vi "Label_Ranking_Average_PS.vi"(7 "Type y_true":T1(ring), 8 "error in (no error)":errorcluster caption="entrée d'erreur (pas d'erreur)", 9 "y_score":string[][](array[string]), 10 "y_true":string[][](array[string]), 11 "label_ranking_average_precision_score":cluster{"sample_weight":dbl[]}) -> (0 "error out":errorcluster caption="sortie d'erreur", 3 "Score":string)   [LabVIEW 2020]
doc: "Compute ranking-based average precision\n\nLabel ranking average precision (LRAP) is the average over each ground truth label assigned to each sample, of the ratio of true vs. total labels with lower score.\n\nThis metric is used in multilabel ranking problem, where the goal is to give better rank to the labels associated to each sample.\n\nThe obtained score is always strictly greater than 0 and the best value is 1.\n\n\n\nParameters : \n\n- y_true : array or sparse matrix, shape = [n_samples, n_labels]\nTrue binary labels in binary indicator format.\n\n- y_score : array, shape = [n_samples, n_labels]\nTarget scores, can either be probability estimates of the positive class, confidence values, or non-thresholded measure of decisions (as returned by “decision_function” on some classifiers).\n\n- sample_weight : array-like of shape (n_samples,), default=None\nSample weights.\n\n\nReturns : \n\n- score : float"
uses:
  Label_Ranking_Average_PS.lvclass
panel:
  out "Label_Ranking_Average_PS en entrée":refnum<class "Label_Ranking_Average_PS.lvclass">
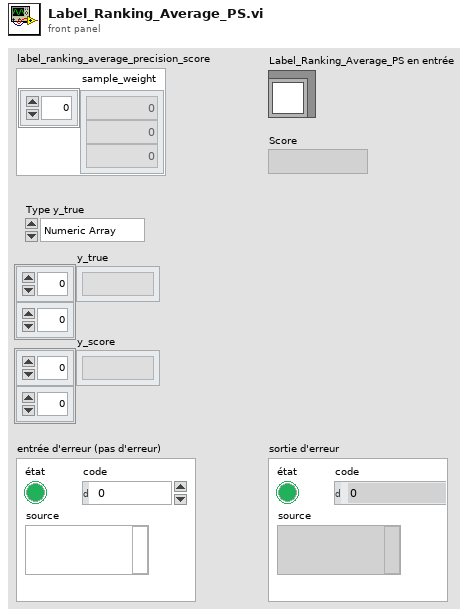
[diagram p1: front panel]
types:
  T1 = enum16{"Numeric Array", "String Array", "Sparse"}
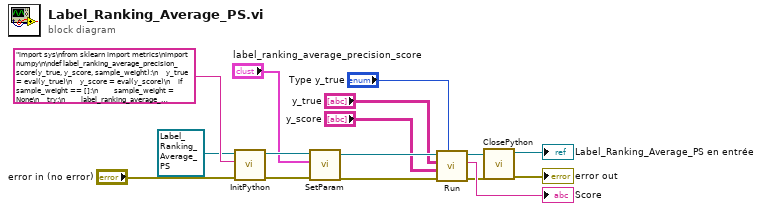
[diagram p0: block diagram]
diagram:
  n1 = call-dynamic "InitPython.vi"("error in (no error)"="error in (no error)", "Python Instruction"="import sys\nfrom sklearn import metrics\nimport numpy\n\ndef label_ranking_average_precision_score(y_true, y_score, sample_weight):\n    y_true = eval(y_true)\n    y_score = eval(y_score)\n    if sample_weight == []:\n        sample_weight = None\n    try:\n        label_ranking_average_precision_score = metrics.label_ranking_average_precision_score(y_true, y_score, sample_weight)\n        label_ranking_average_precision_score = label_ranking_average_precision_score.tolist()\n        return str(label_ranking_average_precision_score)\n    except:\n        erreur = sys.exc_info()\n        typerr = u\"%s\" % (erreur[0])\n        typerr = typerr[typerr.find(\"'\")+1:typerr.rfind(\"'\")]\n        msgerr = u\"%s\" % (erreur[1])\n        message = str('/!\\\\ {0} : {1}'. format(typerr,msgerr))\n        return message", "Scikit-learn en entrée"=refnum<class "Label_Ranking_Average_PS.lvclass"> refnum ("Label_Ranking_Average_PS.lvclass")) -> ("error out"=w9:errorcluster, "Scikit-learn en sortie"=w11:refnum<class "Label_Ranking_Average_PS.lvclass">)  [unwired: 7 in]
  n2 = call-dynamic "SetParam.vi"("error in (no error)"=w9, "label_ranking_average_precision_score"="label_ranking_average_precision_score", "Label_Ranking_Average_PS in"=w11) -> ("error out"=w7:errorcluster, "Label_Ranking_Average_PS out"=w8:refnum<class "Label_Ranking_Average_PS.lvclass">)  [unwired: 7 in]
  n3 = call-dynamic "Run.vi"("Type y_true"="Type y_true", "error in (no error)"=w7, "y_score"="y_score", "y_true"="y_true", "Label_Ranking_Average_PS en entrée"=w8) -> ("error out"=w4:errorcluster, "String Data"=→"Score":string, "Label_Ranking_Average_PS en entrée"=w6:refnum<class "Label_Ranking_Average_PS.lvclass">)  [unwired: 4 in]
  n4 = call-dynamic "ClosePython.vi"("error in (no error)"=w4, "Scikit-learn en entrée"=w6) -> ("error out"=→"error out":errorcluster, "Scikit-learn en sortie"=→"Label_Ranking_Average_PS en entrée":refnum<class "Label_Ranking_Average_PS.lvclass">)  [unwired: 8 in]
